vi "Culver Drive.vi"(7 "Toggle R":bool, 8 "Sensitivity":ext format="%#.6f", 10 "Y":dbl(knob) step=0.1 scale=-1.0..1.0, 11 "X":dbl(knob) step=0.1 scale=-1.0..1.0) -> (3 "R":ext)   [LabVIEW 2014]
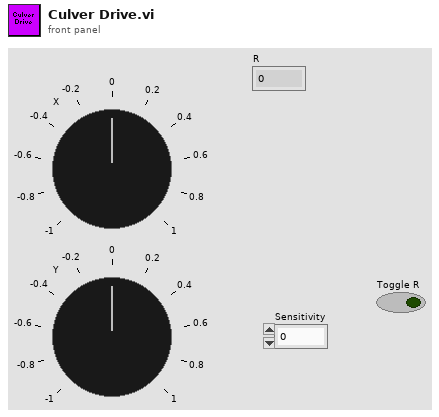
[diagram p1: front panel]
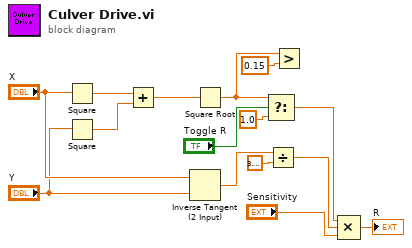
[diagram p0: block diagram]
diagram:
  n1 = Square(x="X") -> (x^2=w13:dbl)
  n2 = Square(x="Y") -> (x^2=w14:dbl)
  n3 = Add(x=w13, y=w14) -> (x+y=w12:dbl)
  n4 = Inverse Tangent (2 Input)(1:"Y", 2:"X") -> (0:w10:dbl)
  n5 = Square Root(x=w12) -> (sqrt(x)=w2:dbl)
  n6 = Select(t=w2, s="Toggle R", f=1.0) -> (s? t:f=w5:dbl)
  n7 = Divide(x=w10, y=3.141592653589793) -> (x/y=w9:dbl)
  n8 = Greater?(x=w2, y=0.15) -> ()  [unwired: 1 out]
  n9 = Compound Arithmetic op=MULTIPLY(w5, w9, "Sensitivity") -> (→"R":ext)
